vi "Build Log Message.vi"(8 "error in":errorcluster, 9 "Message":string, 10 "Level":enum16{"Error", "Warning", "Info", "Debug"}(ring), 11 "Custom Device Name":string) -> (0 "error out":errorcluster, 3 "Log Message":string)   [LabVIEW 2026, in "Template.lvlib" / "Template.lvclass"]
uses:
  Template.lvclass
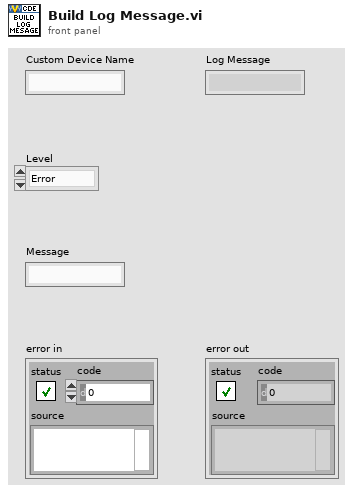
[diagram p1: front panel]
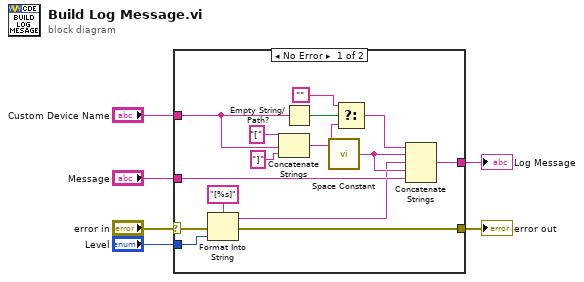
[diagram p0: block diagram]
diagram:
  n1 = case shown="No Error" "error in" {
    selector: "error in" -> [w21 w23]
    tunnel: "Custom Device Name" -> [w11 _]
    tunnel: "Level" -> [w10 _]
    tunnel: "Message" -> [w9 w22]
    tunnel: [w8 w22] -> w1
    tunnel: [w20 w23] -> w5
    frame No Error {
      n2 = Format Into String(format string="[%s]", error in=w21, w10) -> (resulting string=w7:string, error out=w20:errorcluster)  [unwired: 1 in]
      n3 = Concatenate Strings("[", w11, "]") -> (w15:string)
      n4 = Empty String/Path?(string/path=w11) -> (empty?=w19:bool)
      n5 = call <vilib>:"Space Constant.vi"() -> ("String"=w12:string)
      n6 = Select(t="", s=w19, f=w15) -> (s? t:f=w13:string)
      n7 = Concatenate Strings(w13, w12, w7, w12, w9) -> (w8:string)
    }
    frame Error {
    }
  }
  "error out" <- w5
  "Log Message" <- w1
